vi "notify_main.vi"() -> ()   [LabVIEW 2023]
panel:
  in  "Array":dbl[](array[numeric])
  in  "Stop Button":bool
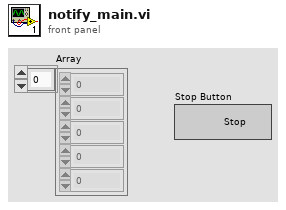
[diagram p1: front panel]
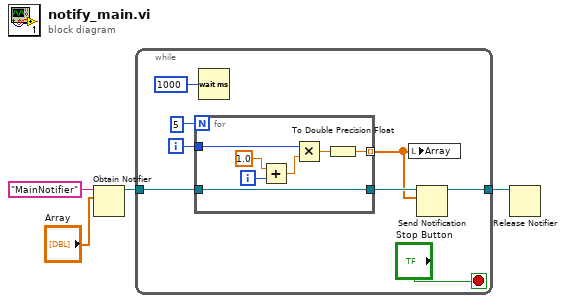
[diagram p0: block diagram]
diagram:
  n1 = Obtain Notifier(name (unnamed)="MainNotifier", notification data type="Array") -> (notifier out=w3:refnum<notifier>)  [unwired: 2 in, 2 out]
  n2 = while {
    tunnel: w3 -> [w7]
    tunnel: [w10] -> w2
    i -> [w8]
    stop <- "Stop Button" stop-if-true
    n3 = for {
      N: 5 -> [_]
      tunnel: w8 -> [w19]
      tunnel: [w16] -> w5 mode=indexing
      tunnel: w7 -> [w18]
      tunnel: [w18] -> w6
      i -> [w13]
      n4 = Add(x=1.0, y=w13) -> (x+y=w15:dbl)
      n5 = Multiply(x=w19, y=w15) -> (x*y=w17:dbl)
      n6 = To Double Precision Float(number=w17) -> (double precision float=w16:dbl)
    }
    n7 = Wait (ms)(milliseconds to wait=u32 1000) -> ()  [unwired: 1 out]
    n8 = local write "Array"(w5) -> ()
    n9 = Send Notification(notification=w5, notifier=w6) -> (notifier out=w10:refnum<notifier>)  [unwired: 1 in, 1 out]
  }
  n10 = Release Notifier(notifier=w2) -> ()  [unwired: 2 in, 3 out]
